vi "Main.vi"(8 "Right Result":bool, 10 "State":T1, 11 "Data":bool[](array[boolean])=[FALSE, FALSE, FALSE, FALSE, FALSE, FALSE, FALSE, FALSE, FALSE, FALSE, FALSE, FALSE, FALSE, FALSE, FALSE]) -> (3 "Coefficients":u16[](array[numeric]))   [LabVIEW 2015]
uses:
  StateCASEType.ctl
  <vilib>/rvi/Emulation/niFpgaGetClockAttributes.vi
  <vilib>/rvi/Emulation/niFpgaSctlEmulationGetInTimedLoop.vi
  <vilib>/rvi/Emulation/niFpgaEmulationReportErrorSimple.vi
  <vilib>/rvi/Emulation/niFpgaProcessEmulError.vi
  <vilib>/rvi/eio/common/nirviEmuTemplateMethod_errors.vi
  <vilib>/rvi/Emulation/niFpgaCriticalErrorInLSC.vi
  <vilib>/eio/EIONode/EIONode.xnode
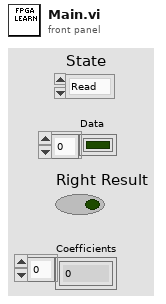
[diagram p1: front panel]
types:
  T1 = typedef "StateCASEType.ctl" = enum16{"Read", "Idle", "Execute", "End"}
  T2 = cluster{"Data[0]":bool, "Data[1]":bool, "Data[2]":bool, "Data[3]":bool, "Data[4]":bool, "Data[5]":bool, "Data[6]":bool, "Data[7]":bool, "Data[8]":bool, "Data[9]":bool, "Data[10]":bool, "Data[11]":bool, "Data[12]":bool, "Data[13]":bool, "Data[14]":bool}
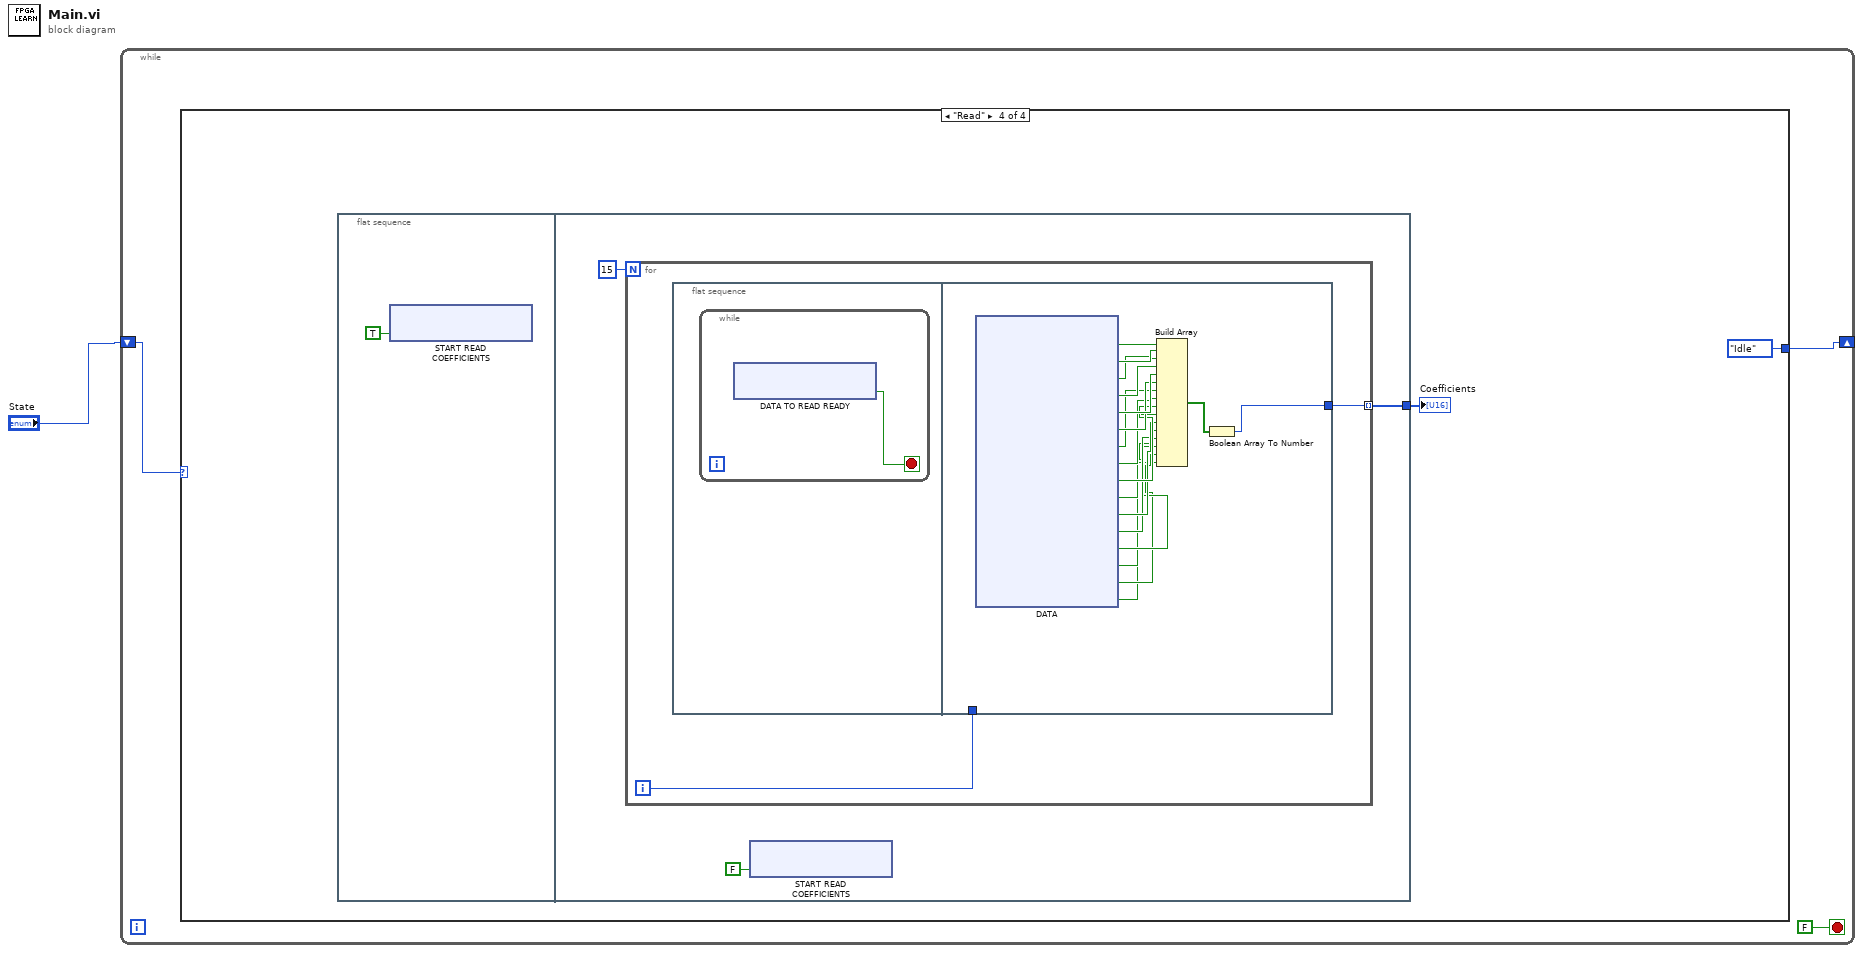
[diagram p0: block diagram]
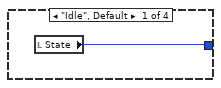
[diagram p2: hidden frame]
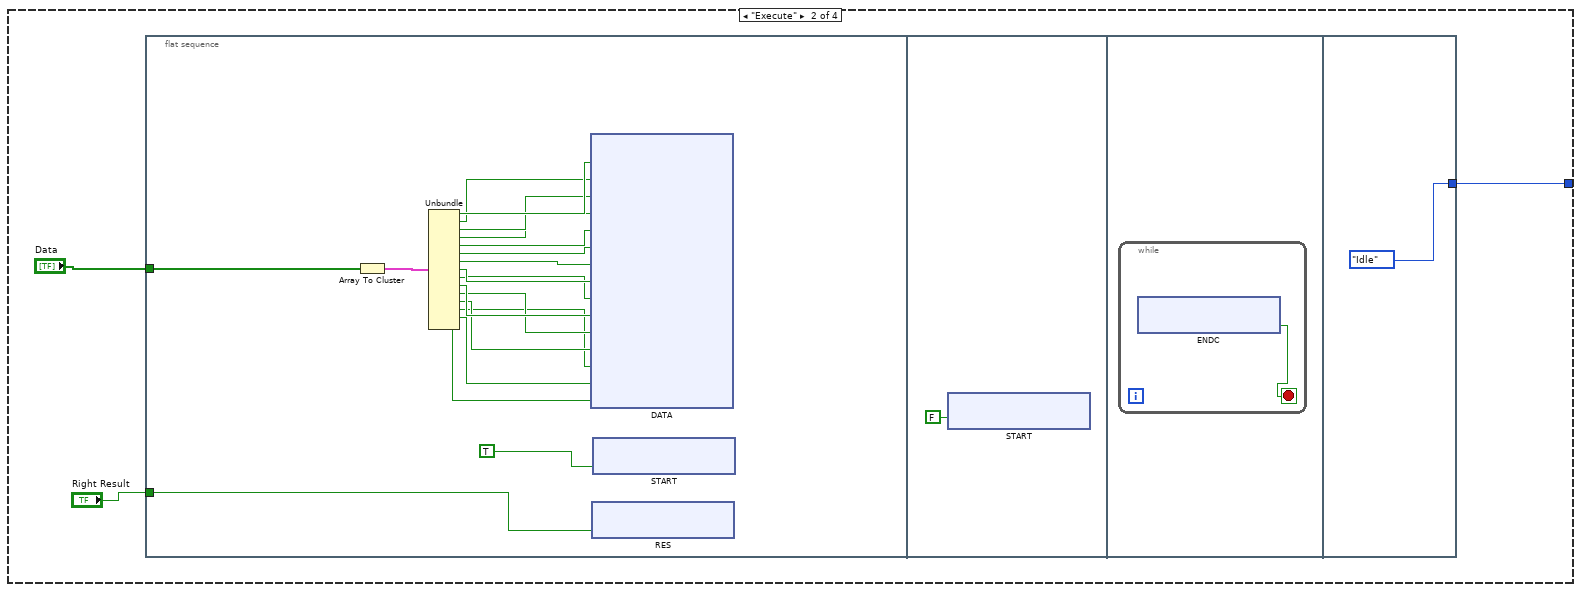
[diagram p3: hidden frame]
diagram:
  n1 = while {
    shift-right: [w4] -> _
    shift-left: "State" -> [w2]
    stop <- FALSE stop-if-true
    n2 = case shown="\"Read\"" w2 {
      selector: w2 -> [_ _ w31 _]
      tunnel: [w5 w6 w31 StateCASEType."Idle" ("State")] -> w4
      frame "Idle", Default {
        n3 = local read "State"() -> (w5:T1)
      }
      frame "Execute" {
        n4 = flat-sequence {
          tunnel: "Right Result" -> [w10]
          tunnel: "Data" -> [w9]
          tunnel: [StateCASEType."Idle" ("State")] -> w6
          frame #0 {
            n5 = Array To Cluster(array=w9) -> (cluster=w27:T2)
            n6 = Unbundle(w27) -> ("Data[0]"=w26:bool, "Data[1]"=w25:bool, "Data[2]"=w24:bool, "Data[3]"=w23:bool, "Data[4]"=w22:bool, "Data[5]"=w21:bool, "Data[6]"=w20:bool, "Data[7]"=w19:bool, "Data[8]"=w18:bool, "Data[9]"=w17:bool, "Data[10]"=w16:bool, "Data[11]"=w15:bool, "Data[12]"=w14:bool, "Data[13]"=w13:bool, "Data[14]"=w12:bool)
            n7 = xnode "DATA"("Connector1/DIO0"=w26, "Connector1/DIO1"=w25, "Connector1/DIO2"=w24, "Connector1/DIO3"=w23, "Connector1/DIO4"=w22, "Connector1/DIO5"=w21, "Connector1/DIO6"=w20, "Connector1/DIO7"=w19, "Connector1/DIO8"=w18, "Connector1/DIO9"=w17, "Connector1/DIO10"=w16, "Connector1/DIO11"=w15, "Connector1/DIO12"=w14, "Connector1/DIO13"=w13, "Connector1/DIO14"=w12) -> ()  [unwired: 15 in, 15 out]
            n8 = xnode "RES"("Connector1/DIO31"=w10) -> ()  [unwired: 1 in, 1 out]
            n9 = xnode "START"("Connector1/DIO30"=TRUE) -> ()  [unwired: 1 in, 1 out]
          }
          frame #1 {
            n10 = xnode "START"("Connector1/DIO30"=FALSE) -> ()  [unwired: 1 in, 1 out]
          }
          frame #2 {
            n11 = while {
              stop <- w29 stop-if-true
              n12 = xnode "ENDC"() -> ("Connector1/DIO26"=w29:bool)  [unwired: 1 in, 1 out]
            }
          }
          frame #3 {
          }
        }
      }
      frame "End" {
      }
      frame "Read" {
        n13 = flat-sequence {
          tunnel: [w36] -> w32
          frame #0 {
            n14 = xnode "START READ COEFFICIENTS"("Connector1/DIO38"=TRUE) -> ()  [unwired: 1 in, 1 out]
          }
          frame #1 {
            n15 = for {
              N: 15 -> [_]
              tunnel: [w38] -> w36 mode=indexing
              i -> [w39]
              n16 = flat-sequence {
                tunnel: w39 -> [_]
                tunnel: [w41] -> w38
                frame #0 {
                  n17 = while {
                    stop <- w40 stop-if-true
                    n18 = xnode "DATA TO READ READY"() -> ("Connector1/DIO39"=w40:bool)  [unwired: 1 in, 1 out]
                  }
                }
                frame #1 {
                  n19 = xnode "DATA"() -> ("Connector2/DIO0"=w58:bool, "Connector2/DIO1"=w57:bool, "Connector2/DIO2"=w56:bool, "Connector2/DIO3"=w55:bool, "Connector2/DIO4"=w54:bool, "Connector2/DIO5"=w53:bool, "Connector2/DIO6"=w52:bool, "Connector2/DIO7"=w51:bool, "Connector2/DIO8"=w50:bool, "Connector2/DIO9"=w49:bool, "Connector2/DIO10"=w48:bool, "Connector2/DIO11"=w47:bool, "Connector2/DIO12"=w46:bool, "Connector2/DIO13"=w45:bool, "Connector2/DIO14"=w44:bool, "Connector2/DIO15"=w43:bool)  [unwired: 16 in, 16 out]
                  n20 = Build Array(w58, w57, w56, w55, w54, w53, w52, w51, w50, w49, w48, w47, w46, w45, w44, w43) -> (w42:bool[])
                  n21 = Boolean Array To Number(Boolean array=w42) -> (number=w41:u16)
                }
              }
            }
            n22 = xnode "START READ COEFFICIENTS"("Connector1/DIO38"=FALSE) -> ()  [unwired: 1 in, 1 out]
          }
        }
        "Coefficients" <- w32
      }
    }
  }
